vi "CreateListenerProcess.vi"(8 "error in (no error)":errorcluster, 9 "master":bool, 10 "process name":string, 11 "Qbus in":refnum<class "Qbus.lvclass">) -> (0 "error in (no error)":errorcluster, 3 "Qbus out":refnum<class "Qbus.lvclass">)   [LabVIEW 2017, in "Qbus.lvclass"]
doc: "Integrates the specified process with the Qbus message bus."
uses:
  <vilib>/addons/Qbus/Qbus.lvclass
  <vilib>/addons/Qbus/Qbus.lvclass/Qbus.ctl
  <vilib>/addons/Qbus/controls/message.ctl
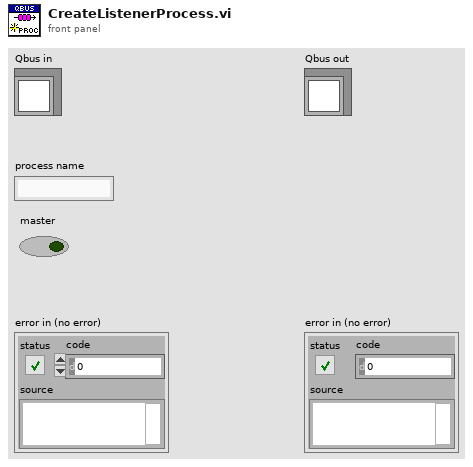
[diagram p1: front panel]
types:
  T1 = typedef "Qbus.lvclass/message.ctl" = cluster{"MsgName":string, "MsgValue":variant}
  T2 = typedef "Qbus.lvclass/data.ctl" = cluster{"Queues":variant, "Subscriptions":variant, "MasterQ":string}
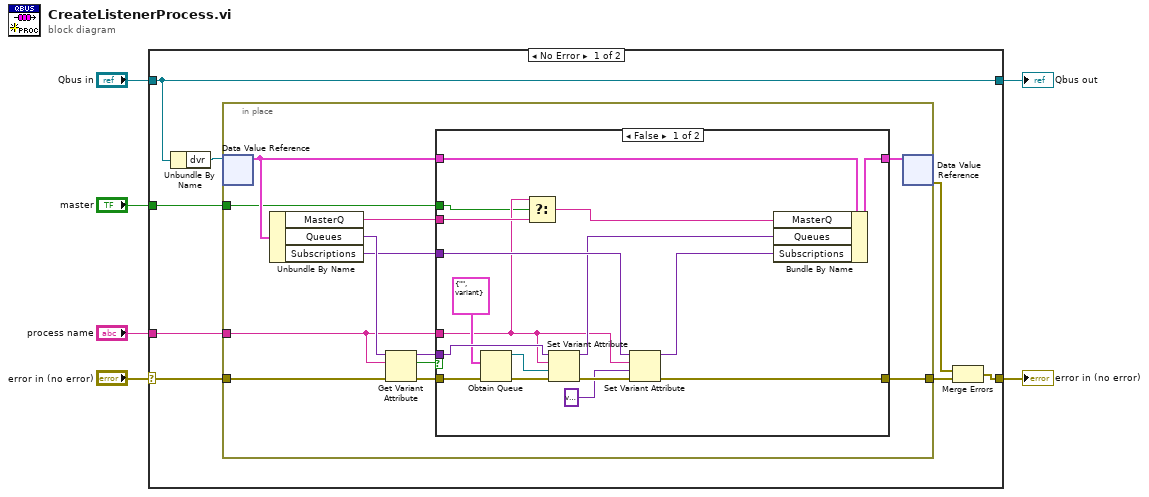
[diagram p0: block diagram]
diagram:
  n1 = case shown="No Error" "error in (no error)" {
    selector: "error in (no error)" -> [w10 w47]
    tunnel: [w9 w47] -> w5
    tunnel: [w14 w46] -> w3
    tunnel: "Qbus in" -> [w14 w46]
    tunnel: "process name" -> [w12 _]
    tunnel: "master" -> [w7 _]
    frame No Error {
      n2 = Unbundle By Name(w14) -> ("dvr"=w13:refnum<data-value>)
      n3 = in-place {
        in-place-border: w10 -> [w26]
        in-place-border: w12 -> [w18]
        in-place-border: [w17] -> w8
        in-place-border: w7 -> [w15]
        n4 = in-place-dvr #1(w13) -> (w22:T2)  [unwired: 1 out]
        n5 = Unbundle By Name(w22) -> ("MasterQ"=w16:string, "Queues"=w21:variant, "Subscriptions"=w19:variant)
        n6 = Get Variant Attribute(Variant=w21, name=w18, error in=w26) -> (duplicate Variant=w20:variant, found=w25:bool, error out=w24:errorcluster)  [unwired: 1 in, 1 out]
        n7 = case shown="False" w25 {
          tunnel: w24 -> [w36 w44]
          tunnel: [w42 w45] -> w23
          tunnel: w22 -> [w43 w45]
          tunnel: w20 -> [w41 _]
          tunnel: w19 -> [w40 _]
          tunnel: w18 -> [w30 _]
          tunnel: [w27 w44] -> w17
          tunnel: w16 -> [w31 _]
          tunnel: w15 -> [w29 _]
          frame False {
            n8 = Obtain Queue(element data type=T1 {"MsgName"="", "MsgValue"=variant} ("Message"), error in (no error)=w36) -> (queue out=w34:refnum<queue>, error out=w35:errorcluster)  [unwired: 3 in, 1 out]
            n9 = Select(t=w30, s=w29, f=w31) -> (s? t:f=w28:string)
            n10 = Set Variant Attribute(Variant=w41, name=w30, value=w34, error in=w35) -> (Variant out=w38:variant, error out=w39:errorcluster)  [unwired: 1 out]
            n11 = Set Variant Attribute(Variant=w40, name=w30, value=variant ("Subscriptions"), error in=w39) -> (Variant out=w37:variant, error out=w27:errorcluster)  [unwired: 1 out]
            n12 = Bundle By Name(cluster=w43, "MasterQ"=w28, "Queues"=w38, "Subscriptions"=w37) -> (w42:T2)
          }
          frame True {
          }
        }
        n13 = in-place-dvr #1(w23) -> (w11:errorcluster)  [unwired: 1 out]
      }
      n14 = Merge Errors(w11, w8) -> (w9:errorcluster)
    }
    frame Error {
    }
  }
  "error in (no error)" <- w5
  "Qbus out" <- w3
